vi "Get or Create Response.vi"(8 "Error In":errorcluster, 11 "Message Refnum In":T1 format="%.0x") -> (0 "Error Out":errorcluster, 2 "Response Refnum":T1=18446744073709551615 format="%.0x", 3 "Message Refnum Out":T1=18446744073709551615 format="%.0x")   [LabVIEW 2020, in "Instrument Addon Scripting API.lvlib"]
uses:
  Instrument Addon Scripting API.lvlib
  <vilib>/NI VeriStand/Custom Device API/Custom Device Item Ref.ctl
  Shared Directory/Constants.vi
  <vilib>/NI VeriStand/Custom Device Tools/Custom Device Utility Library/NI VeriStand - Search for Item by GUID.vi
  Shared Directory/Instrument Addon Shared.lvlib
  <vilib>/NI VeriStand/Custom Device Tools/Custom Device Utility Library/Custom Device Utility Library.lvlib
  <vilib>/NI VeriStand/Custom Device API/Custom Device API.lvlib
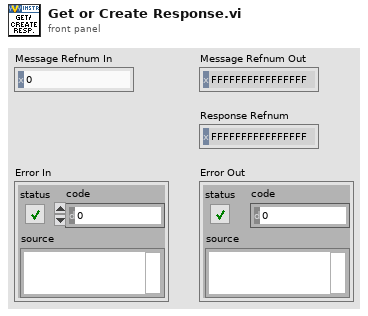
[diagram p1: front panel]
types:
  T1 = typedef "Custom Device API.lvlib/Custom Device Item Ref.ctl" = u64
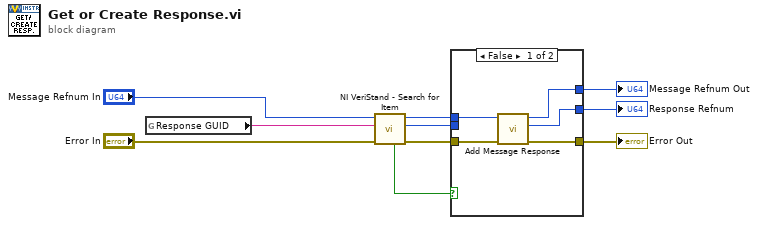
[diagram p0: block diagram]
diagram:
  n1 = global read "Constants.vi" "Response GUID"() -> (w2:string)
  n2 = call-poly <vilib>:"NI VeriStand - Search for Item.vi"("error in"="Error In", "Item GUID"=w2, "Section Ref in"="Message Refnum In") -> ("error out"=w9:errorcluster, "Item Ref"=w6:T1, "Section Ref out"=w5:T1, "Found"=w4:bool)  [unwired: 5 in]
  n3 = case shown="False" w4 {
    tunnel: w5 -> [w14 w17]
    tunnel: w6 -> [_ w18]
    tunnel: [w11 w18] -> w7
    tunnel: [w13 w17] -> w8
    tunnel: w9 -> [w15 w16]
    tunnel: [w12 w16] -> w10
    frame False {
      n4 = call "Add Message Response.vi"("Error In"=w15, "Message Refnum In"=w14) -> ("Error Out"=w12:errorcluster, "Response Section Ptr"=w11:T1, "Message Refnum Out"=w13:T1)  [unwired: 7 in]
    }
    frame True {
    }
  }
  "Response Refnum" <- w7
  "Message Refnum Out" <- w8
  "Error Out" <- w10
